vi "Page Number Formatted string.vi"(0 "Page #":i32, 2 "Character type":T1=enum."ASCII", 5 "Start with #":i32, 7 "Total page #":i32, 9 "Start at page":i32, 11 "Page # cluster":T2) -> (4 "Temporaty Cell":string, 8 "Page string":string, 15 "Final Cell":string)   [LabVIEW 2019, in "Exaprom PDF.lvlib"]
doc: "Version 2.0\nDeveloped by Jean-Marc Simard\nCopyright © 2012, Exaprom Inc.\nAll rights reserved.\nLicense: BSD"
uses:
  Controls/Header, Footer and Watermark Controls/Page number.ctl
  Controls/Text Controls/Unicode/Type and run direction.ctl
  Exaprom PDF.lvlib
panel:
  # "Y"
  # "X"
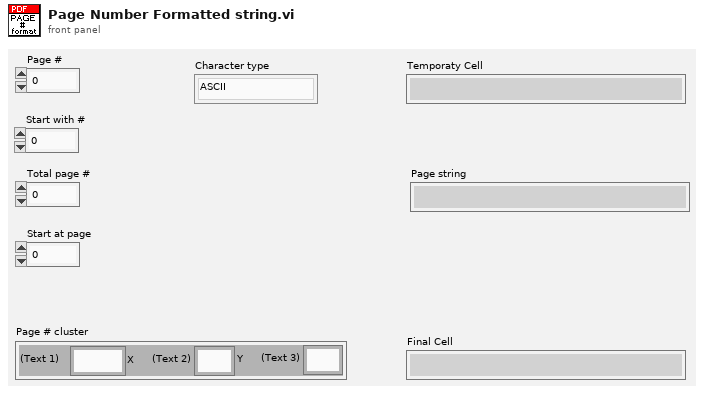
[diagram p1: front panel]
types:
  T1 = typedef "Exaprom PDF.lvlib/Type and run direction.ctl" = enum16{"Select", "ASCII", "UTF-16", "UTF-16 (default)", "UTF-16 (LTR)", "UTF-16 (RTL)"}
  T2 = typedef "Exaprom PDF.lvlib/Page number.ctl" = cluster{"Text 1":string, "Text 2":string, "Text 3":string}
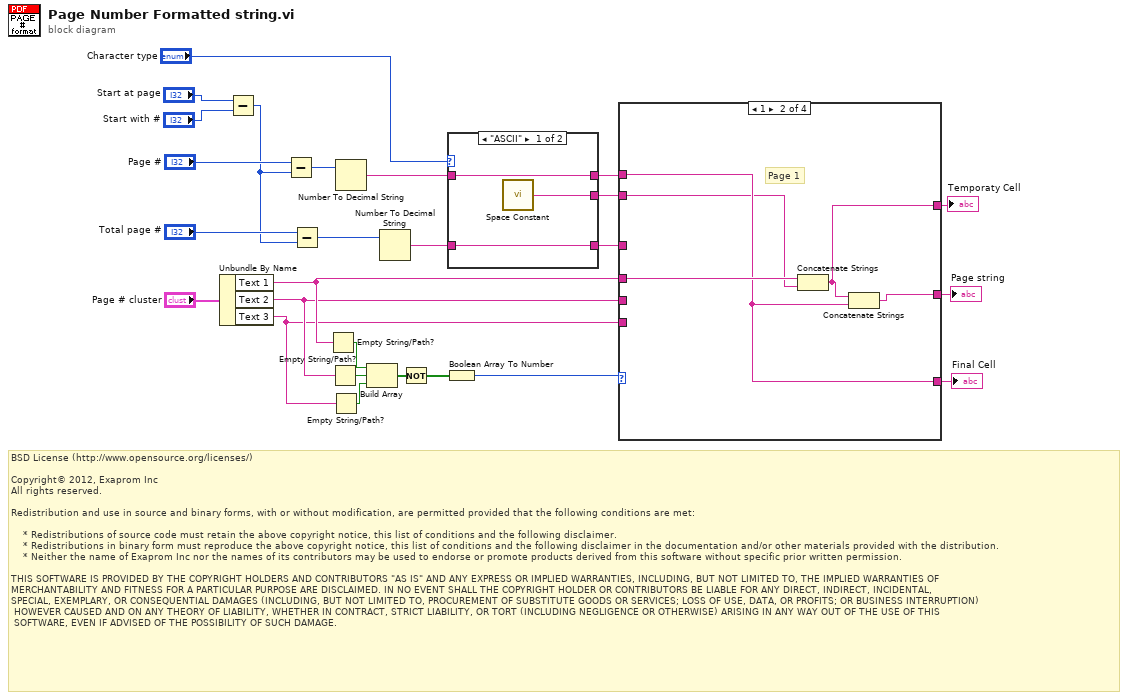
[diagram p0: block diagram]
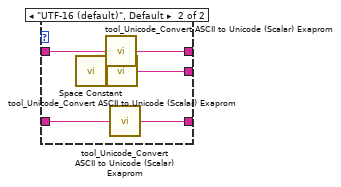
[diagram p2: hidden frame]
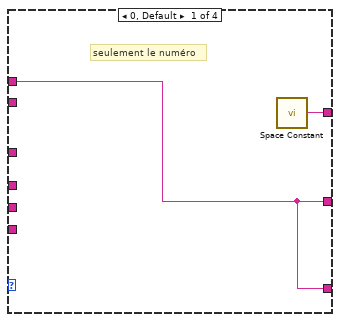
[diagram p3: hidden frame]
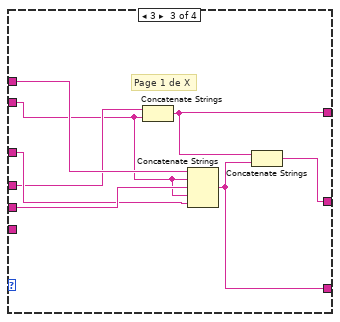
[diagram p4: hidden frame]
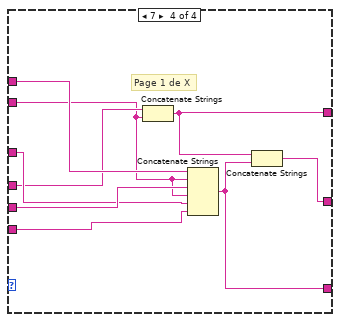
[diagram p5: hidden frame]
diagram:
  # "BSD License (http://www.opensource.org/licenses/)\n\nCopyright© 2012, Exaprom Inc\nAll rights reserved.\n\nRedistribution and use in source and binary forms, with or without modification, are permitted provided that the following conditions are met:\n\n    * Redistributions of source code must retain the above copyright notice, this list of conditions and the following disclaimer.\n    * Redistributions in binary form must reproduce the above copyright notice, this list of conditions and the following disclaimer in the documentation and/or other materials provided with the distribution.\n    * Neither the name of Exaprom Inc nor the names of its contributors may be used to endorse or promote products derived from this software without specific prior written permission.\n\nTHIS SOFTWARE IS PROVIDED BY THE COPYRIGHT HOLDERS AND CONTRIBUTORS \"AS IS\" AND ANY EXPRESS OR IMPLIED WARRANTIES, INCLUDING, BUT NOT LIMITED TO, THE IMPLIED WARRANTIES OF \nMERCHANTABILITY AND FITNESS FOR A PARTICULAR PURPOSE ARE DISCLAIMED. IN NO EVENT SHALL THE COPYRIGHT HOLDER OR CONTRIBUTORS BE LIABLE FOR ANY DIRECT, INDIRECT, INCIDENTAL,\nSPECIAL, EXEMPLARY, OR CONSEQUENTIAL DAMAGES (INCLUDING, BUT NOT LIMITED TO, PROCUREMENT OF SUBSTITUTE GOODS OR SERVICES; LOSS OF USE, DATA, OR PROFITS; OR BUSINESS INTERRUPTION)\n HOWEVER CAUSED AND ON ANY THEORY OF LIABILITY, WHETHER IN CONTRACT, STRICT LIABILITY, OR TORT (INCLUDING NEGLIGENCE OR OTHERWISE) ARISING IN ANY WAY OUT OF THE USE OF THIS\n SOFTWARE, EVEN IF ADVISED OF THE POSSIBILITY OF SUCH DAMAGE."
  n1 = Unbundle By Name("Page # cluster") -> ("Text 1"=w19:string, "Text 2"=w18:string, "Text 3"=w17:string)
  n2 = Subtract(x="Start at page", y="Start with #") -> (x-y=w6:i32)
  n3 = Subtract(x="Page #", y=w6) -> (x-y=w10:i32)
  n4 = Subtract(x="Total page #", y=w6) -> (x-y=w7:i32)
  n5 = Empty String/Path?(string/path=w19) -> (empty?=w25:bool)
  n6 = Empty String/Path?(string/path=w18) -> (empty?=w24:bool)
  n7 = Empty String/Path?(string/path=w17) -> (empty?=w23:bool)
  n8 = Number To Decimal String(number=w10) -> (decimal integer string=w15:string)  [unwired: 1 out]
  n9 = Build Array(w25, w24, w23) -> (w22:bool[])
  n10 = Number To Decimal String(number=w7) -> (decimal integer string=w2:string)  [unwired: 1 out]
  n11 = Not(x=w22) -> (.not. x?=w16:bool[])
  n12 = Boolean Array To Number(Boolean array=w16) -> (number=w21:u32)
  n13 = case shown="\"ASCII\"" "Character type" {
    tunnel: w15 -> [w29 w35]
    tunnel: [w29 w34] -> w5
    tunnel: [w28 w32] -> w3
    tunnel: w2 -> [w27 w30]
    tunnel: [w27 w31] -> w1
    frame "ASCII" {
      n14 = call <vilib>:"Space Constant.vi"() -> ("String"=w28:string)
    }
    frame "UTF-16 (default)", Default {
      n15 = call <vilib>:"Space Constant.vi"() -> ("String"=w33:string)
      n16 = call "tool_Unicode_Convert ASCII to Unicode (Scalar) Exaprom.vi"("ASCII"=w35) -> ("Unicode"=w34:string)  [unwired: 4 in]
      n17 = call "tool_Unicode_Convert ASCII to Unicode (Scalar) Exaprom.vi"("ASCII"=w33) -> ("Unicode"=w32:string)  [unwired: 4 in]
      n18 = call "tool_Unicode_Convert ASCII to Unicode (Scalar) Exaprom.vi"("ASCII"=w30) -> ("Unicode"=w31:string)  [unwired: 4 in]
    }
  }
  n19 = case shown="1" w21 {
    tunnel: w19 -> [_ w42 w47 w56]
    tunnel: w18 -> [_ _ w49 w58]
    tunnel: w17 -> [_ _ _ w52]
    tunnel: w5 -> [w37 w39 w50 w59]
    tunnel: w1 -> [_ _ w48 w57]
    tunnel: [w37 w41 w44 w53] -> w14
    tunnel: [w36 w40 w46 w55] -> w13
    tunnel: [w37 w39 w45 w54] -> w12
    tunnel: w3 -> [_ w38 w43 w51]
    frame 0, Default {
      # "seulement le numéro"
      n20 = call <vilib>:"Space Constant.vi"() -> ("String"=w36:string)
    }
    frame 1 {
      # "Page 1"
      n21 = Concatenate Strings(w42, w38) -> (w40:string)
      n22 = Concatenate Strings(w40, w39) -> (w41:string)
    }
    frame 3 {
      # "Page 1 de X"
      n23 = Concatenate Strings(w47, w43) -> (w46:string)
      n24 = Concatenate Strings(w50, w43, w49, w43, w48) -> (w45:string)
      n25 = Concatenate Strings(w46, w45) -> (w44:string)
    }
    frame 7 {
      # "Page 1 de X"
      n26 = Concatenate Strings(w56, w51) -> (w55:string)
      n27 = Concatenate Strings(w59, w51, w58, w51, w57, w52) -> (w54:string)
      n28 = Concatenate Strings(w55, w54) -> (w53:string)
    }
  }
  "Page string" <- w14
  "Temporaty Cell" <- w13
  "Final Cell" <- w12
